vi "Xbox1ControllerScaler.vi"(11 "DriveJoystickButtonMapping":T1) -> (3 "Speed":dbl)   [LabVIEW 2019]
uses:
  Controls/DriveJoystickData.ctl
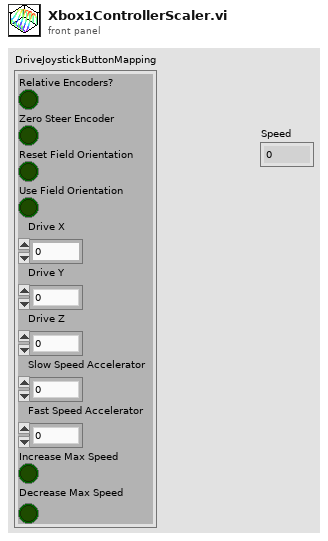
[diagram p1: front panel]
types:
  T1 = typedef "DriveJoystickData.ctl" = cluster{"Relative Encoders?":bool, "Zero Steer Encoder":bool, "Reset Field Orientation":bool, "Use Field Orientation":bool, "Drive X":dbl, "Drive Y":dbl, "Drive Z":dbl, "Slow Speed Accelerator":dbl, "Fast Speed Accelerator":dbl, "Increase Max Speed":bool, "Decrease Max Speed":bool}
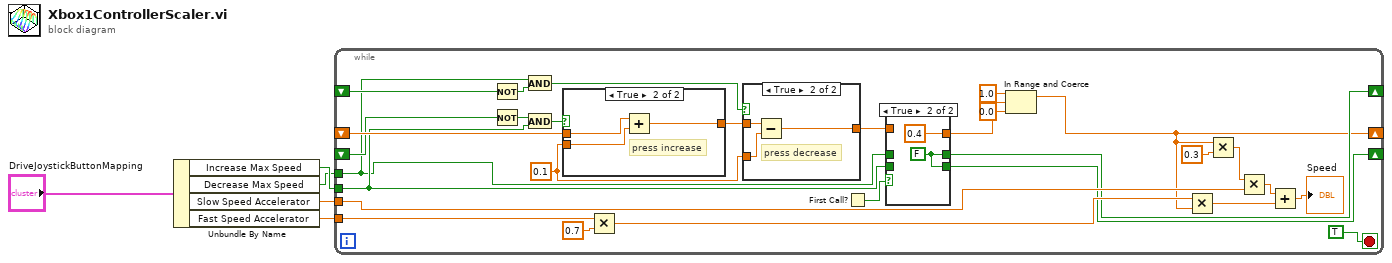
[diagram p0: block diagram]
diagram:
  n1 = Unbundle By Name("DriveJoystickButtonMapping") -> ("Increase Max Speed"=w2:bool, "Decrease Max Speed"=w1:bool, "Slow Speed Accelerator"=w4:dbl, "Fast Speed Accelerator"=w3:dbl)
  n2 = while {
    shift-right: [w6] -> _
    shift-left: _ -> [w21]
    tunnel: w4 -> [w30]
    tunnel: w3 -> [w27]
    shift-right: [w22] -> _
    shift-left: _ -> [w11]
    shift-right: [w23] -> _
    shift-left: _ -> [w19]
    tunnel: w2 -> [w18]
    tunnel: w1 -> [w10]
    stop <- TRUE stop-if-true
    w15 = 0.1 ("x")
    n3 = Not(x=w11) -> (.not. x?=w13:bool)
    n4 = Not(x=w19) -> (.not. x?=w20:bool)
    n5 = And(x=w10, y=w13) -> (x .and. y?=w12:bool)
    n6 = And(x=w20, y=w18) -> (x .and. y?=w14:bool)
    n7 = case shown="True" w14 {
      tunnel: [w39 w41] -> w17
      tunnel: w21 -> [w39 w42]
      tunnel: w15 -> [_ w40]
      frame False {
      }
      frame True {
        # "press increase"
        n8 = Add(x=w42, y=w40) -> (x+y=w41:dbl)
      }
    }
    n9 = Multiply(x=w27, y=0.7) -> (x*y=w28:dbl)
    n10 = case shown="True" w12 {
      tunnel: [w35 w37] -> w16
      tunnel: w17 -> [w35 w38]
      tunnel: w15 -> [_ w36]
      frame False {
      }
      frame True {
        # "press decrease"
        n11 = Subtract(x=w38, y=w36) -> (x-y=w37:dbl)
      }
    }
    n12 = First Call?() -> (First Call?: T/F=w33:bool)
    n13 = case shown="True" w33 {
      tunnel: w16 -> [w45 _]
      tunnel: [w45 0.4] -> w7
      tunnel: w18 -> [w44 _]
      tunnel: w10 -> [w43 _]
      tunnel: [w44 w46] -> w23
      tunnel: [w43 w46] -> w22
      frame False {
      }
      frame True {
        w46 = FALSE
      }
    }
    n14 = In Range and Coerce(upper limit=1.0, x=w7, lower limit=0.0) -> (coerced(x)=w6:dbl)  [unwired: 1 out]
    n15 = Multiply(x=w28, y=w6) -> (x*y=w26:dbl)
    n16 = Multiply(x=w6, y=0.3) -> (x*y=w31:dbl)
    n17 = Multiply(x=w31, y=w30) -> (x*y=w25:dbl)
    n18 = Add(x=w25, y=w26) -> (x+y=→"Speed":dbl)
  }
